vi "Double FFT Mesurament (Max Bin detection - Control - Windowing - DIEGO) test.vi"() -> ()   [LabVIEW 2014]
uses:
  <vilib>/Platform/TimedLoop/XDataNode/timing_clust.ctl
  <vilib>/Platform/TimedLoop/XDataNode/nitl_modes.ctl
  <vilib>/Platform/TimedLoop/XDataNode/wakeup.ctl
  <vilib>/rvi/Analysis/measure/FFT/simModelSupport/niFPGA FFT Streaming Sim Properties.ctl
  <vilib>/rvi/Analysis/measure/FFT/simModelSupport/niFPGA FFT Sim Stream Group Properties.ctl
  <vilib>/rvi/Analysis/measure/FFT/simModelSupport/niFPGA FFT Sim Types.ctl
  <vilib>/rvi/Analysis/measure/FFT/simModelSupport/niFpgaFFTSimArithmeticProperties.ctl
  <vilib>/rvi/Analysis/measure/FFT/simModelSupport/niFpgaFFTSimDfxp.ctl
  <vilib>/fxp/LVFixedPointQuantizationPolicyTypeDef.ctl
  <vilib>/rvi/Analysis/measure/FFT/XNode/niFpgaFFTButterflyDelays.ctl
  <vilib>/rvi/Emulation/niFpgaSctlEmulationGetInTimedLoop.vi
  <vilib>/rvi/Emulation/niFpgaEmulationReportErrorSimple.vi
  <vilib>/rvi/Emulation/niFpgaGetClockAttributes.vi
  <vilib>/rvi/Emulation/niFpgaCriticalErrorInLSC.vi
  <vilib>/rvi/Emulation/niFpgaEmulationIsFPGAContextNoSignature.vi
  <vilib>/rvi/errors/niFpgaSetErrorForExecOnDevCompSimple.vi
  <vilib>/rvi/eio/common/nirviEmuReportErrorAndStop.vi
  <vilib>/rvi/DataTransferAndStorage/Container/Common/niFpgaContainerGetUniqueNameForEmu.vi
  <vilib>/rvi/FIFO/Fifo_Resource/nirvififoEmulationSetSize.vi
  <vilib>/rvi/FIFO/Fifo_Resource/nirviFifoEmulationQueueMgr.vi
  <instcachedir>/0/nirviFifoEmulationQueueMgr_E5CAEC123FF24DC58D834DCA3CDAA9B5.lvgen/nirviFifoEmulationQueueMgr_E5CAEC123FF24DC58D834DCA3CDAA9B5_004.vi
  <vilib>/Utility/error.llb/Clear Errors.vi
  <vilib>/rvi/FIFO/Fifo_Resource/nirvififoEmulationCreateLock.vi
  <vilib>/rvi/Emulation/niFpgaProcessEmulError.vi
  <vilib>/rvi/FIFO/Fifo_Resource/nirvififoEmulationObtainLock.vi
  <vilib>/rvi/FIFO/Fifo_Resource/nirvififoEmulationReleaseLock.vi
  <vilib>/rvi/occurrence/nirviWaitOnOccurrenceBase.vi
  <vilib>/rvi/errors/nirviReportUnexpectedCaseInternalError.vi
  <vilib>/rvi/errors/nirviReportUnexpectedCaseInternalError (U32).vi
  <vilib>/rvi/Memory/Memory_Emulation/niFpgaMemoryEmulationCacheClearOnFirstRun.vi
  <vilib>/rvi/Memory/Memory_Emulation/nirvimemoryEmulationManagerCache_MakeExclusive.vi
  <vilib>/rvi/Memory/Memory_Emulation/niFpgaMemoryEmulationValidateCache.vi
  <vilib>/rvi/Memory/Memory_Emulation/nirvimemoryEmulationManagerCache_InsertValue.vi
  <vilib>/rvi/Memory/Memory_Emulation/nirvimemoryEmulationManagerCache_ReleaseExclusive.vi
  <vilib>/rvi/Memory/Memory_Emulation/nirvimemoryEmulationManagerCache_GetValue.vi
  <vilib>/rvi/Memory/Memory_Emulation/nirvimemoryEmulationManagerCache_SetValue.vi
  <instcachedir>/0/nirviFifoEmulationQueueMgr_E5CAEC123FF24DC58D834DCA3CDAA9B5.lvgen/nirviFifoEmulationQueueMgr_E5CAEC123FF24DC58D834DCA3CDAA9B5_003.vi
  <vilib>/rvi/FIFO/Fifo_Resource/nirvififoEmulationDetermineInputValidOut.vi
  <vilib>/rvi/Memory/Memory_Emulation/nirvimemoryFastEmulation.vi
  <vilib>/rvi/Memory/Memory_Emulation/nirvimemoryEmulation.vi
  <vilib>/rvi/interface/RandomDataEmulation/niFpgaRandomDataHandleErrors.vi
  <vilib>/rvi/Analysis/measure/FFT/simModelSupport/niFpgaFFTSimModelStreamingCore.vi
  <vilib>/rvi/eio/common/nirviEmuTemplateMethod_errors.vi
  <vilib>/Platform/TimedLoop/XDataNode/XDataNode.xnode
  <vilib>/rvi/DataTransferAndStorage/Container/XNode/niFpgaContainer.xnode
  <vilib>/rvi/FIFO/Fifo_Resource/nirvififoEmulationRead.vi
  <vilib>/rvi/DataTransferAndStorage/Register/Emulation/niFpgaRegisterEmulation.vi
  <vilib>/rvi/FIFO/Fifo_Resource/nirvififoEmulationWrite.vi
  <vilib>/rvi/FIFO/Fifo_Resource/nirvififoEmulationGetNumberOfElementsToWrite.vi
  <vilib>/rvi/interface/RandomDataEmulation/nirviRandomDataFpgaReadWriteTemplate.vi
  <vilib>/rvi/Analysis/measure/FFT/XNode/niFpgaFFT.xnode
  <vilib>/eio/EIOMethodNode/EIOMethodNode.xnode
  <vilib>/Platform/TimedLoop/XDataNode/XDNodeRunTimeDep.lvlib
panel:
  in  "snapshot":bool
  in  "first bin":i32=4
  in  "last bin":i32=251
  in  "lower limit 2":u32=682
  in  "lower limit 1":u32=57
  in  "upper limit 2":u32=1194
  in  "upper limit 1":u32=569
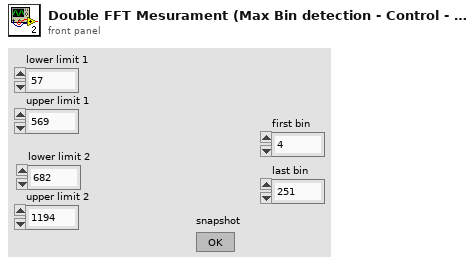
[diagram p1: front panel]
types:
  T1 = typedef "XDNodeRunTimeDep.lvlib/timing_clust.ctl" = cluster{"Expected End [f-1]":u64, "Actual End [f-1]":u64, "Finished Late? [f-1]":bool, "Expected End [i-1]":u64, "Actual End [i-1]":u64, "Finished Late? [i-1]":bool, "Expected Start [i]":u64, "Actual Start [i]":u64, "Expected Start [f]":u64, "Actual Start [f]":u64, "Source Name":string, "Structure Name":string, "Period":i64, "Deadline":i64, "Offset":i64, "Start":i64, "Priority":i32, "Timeout":i32, "Mode":T2, "Wakeup Reason":T3, "Error":errorcluster, "Source Type":string, "Secondary Source Type":string, "Global End Time":u64, "Global Start Time":u64, "Frame Duration":u64, "Iteration Duration":u64, "Assigned CPU":i32, "I/O Scan Engine Mode":u32}
  T2 = typedef "XDNodeRunTimeDep.lvlib/nitl_modes.ctl" = enum32{"No Change", "Process missed periods, maintain original phase", "Discard missed periods, maintain original phase", "Process missed periods, ignore original phase", "Discard missed periods, ignore original phase"}
  T3 = typedef "XDNodeRunTimeDep.lvlib/wakeup.ctl" = enum32{"Normal", "Aborted", "Asynchronous wakeup", "Timing source error", "Timed loop error", "Timeout"}
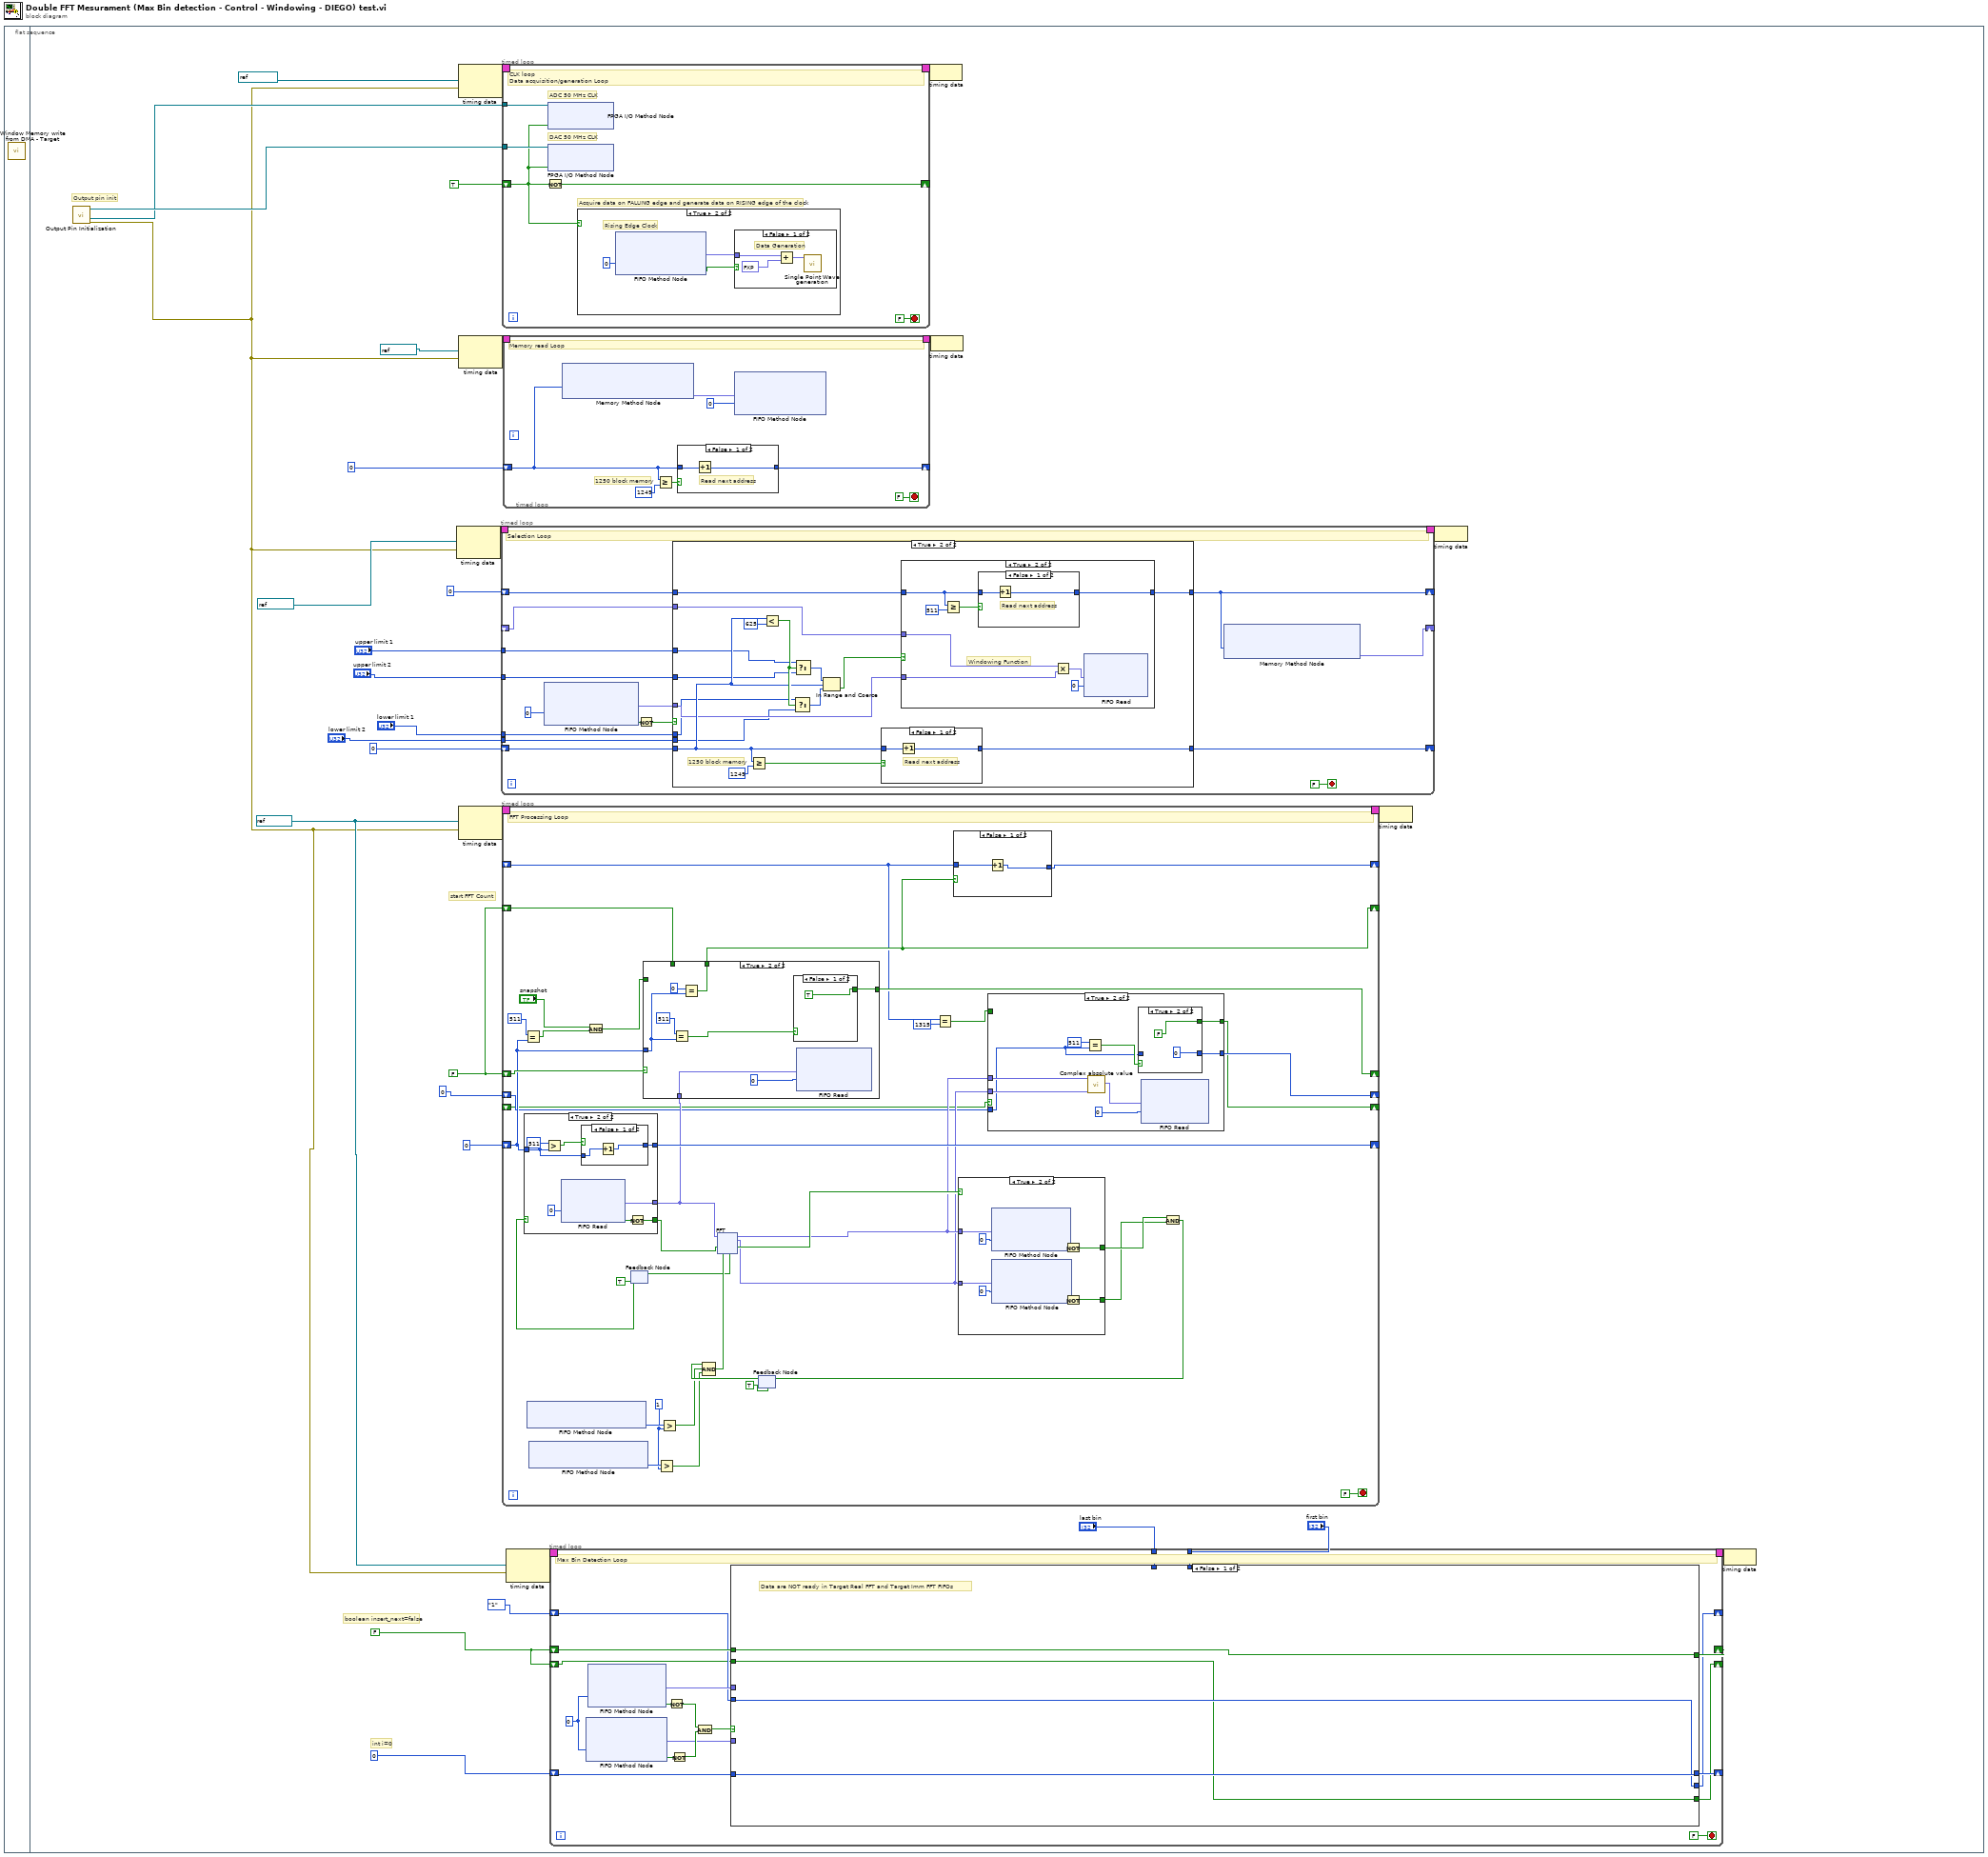
[diagram p0: block diagram]
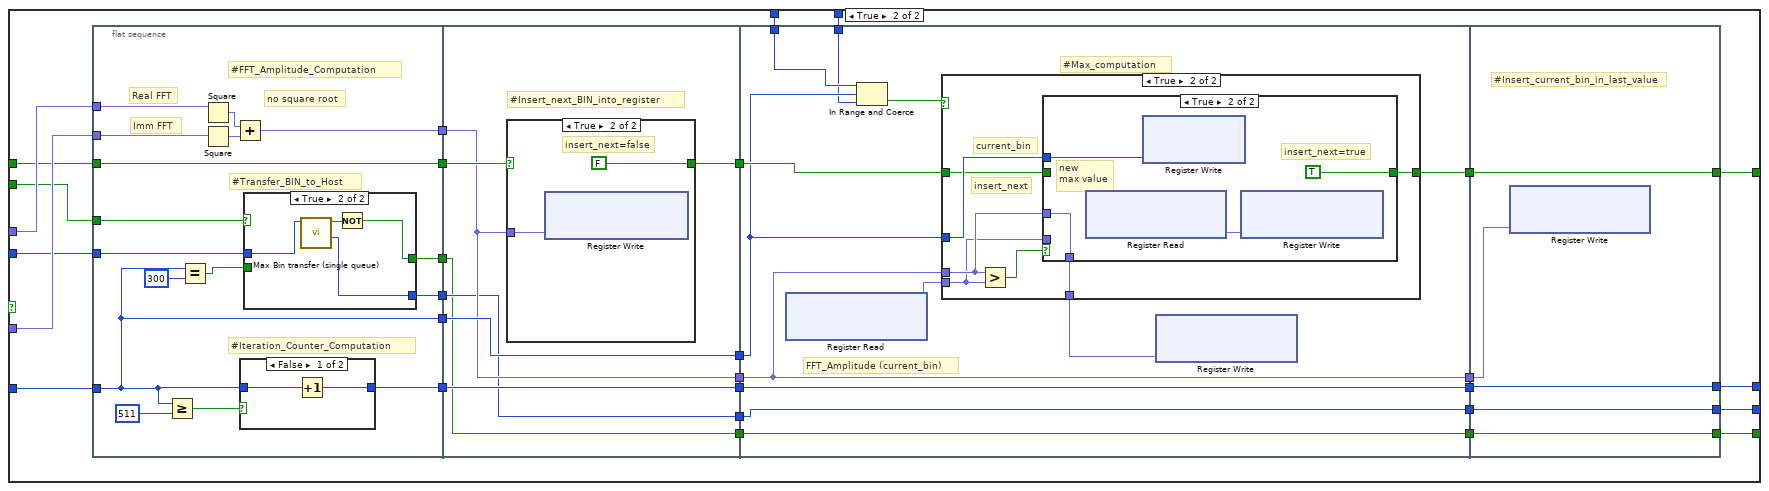
[diagram p2: hidden frame]
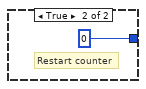
[diagram p4: hidden frame]
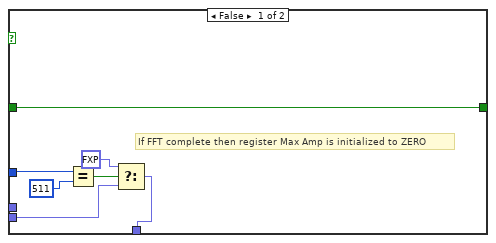
[diagram p6: hidden frame]
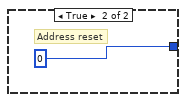
[diagram p10: hidden frame]
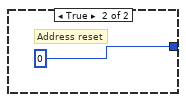
[diagram p11: hidden frame]
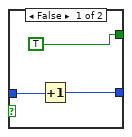
[diagram p13: hidden frame]
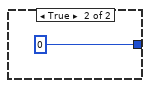
[diagram p14: hidden frame]
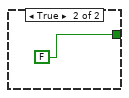
[diagram p16: hidden frame]
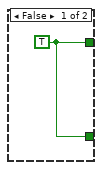
[diagram p17: hidden frame]
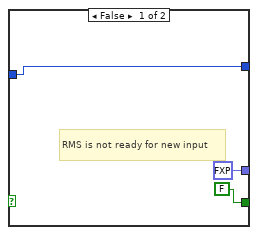
[diagram p18: hidden frame]
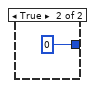
[diagram p19: hidden frame]
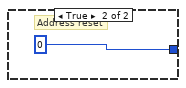
[diagram p20: hidden frame]
diagram:
  n1 = flat-sequence {
    frame #0 {
      n2 = call "Window Memory write from DMA - Target.vi"() -> ()  [unwired: 12 in]
    }
    frame #1 {
      w4 = FALSE
      w1 = FALSE
      w14 = refnum<k21> "50MHz" ("Source Name")
      # "start FFT Count"
      # "int i=0"
      # "boolean insert_next=false"
      # "Output pin init"
      n3 = call "Output Pin Initialization.vi"() -> ("error out"=w13:errorcluster, "I/O Out Clock DAC (pin16)"=w18:refnum<k21>, "I/O Out Clock ADC (pin17)"=w19:refnum<k21>)  [unwired: 8 in]
      n4 = node-c288(refnum<k21> "50MHz" ("Source Name"), w13) -> (w27:T1)
      n5 = node-c288(refnum<k21> "100MHz" ("Source Name"), w13) -> (w33:T1)
      n6 = node-c288(w14, w13) -> (w29:T1)
      n7 = node-c288(refnum<k21> "50MHz" ("Source Name"), w13) -> (w31:T1)
      n8 = timed-loop {
        timing: w27 -> [_]
        timing-out: [_] -> w26
        shift-right: [w178] -> _
        shift-left: u32 0 -> [w177]
        tunnel: "upper limit 1" -> [w172]
        tunnel: "upper limit 2" -> [w171]
        tunnel: "lower limit 1" -> [w170]
        tunnel: "lower limit 2" -> [w169]
        shift-right: [w165] -> _
        shift-left: u32 0 -> [w168]
        shift-right: [w166] -> _
        shift-left: _ -> [w167]
        stop <- FALSE stop-if-true
        # "Selection Loop"
        n9 = xnode ("FIFO Method Node")("Timeout"=0) -> ("Element"=w174:fxp<+/-,12,12>, "Timed Out?"=w175:bool)  [unwired: 1 in, 1 out]
        n10 = Not(x=w175) -> (.not. x?=w176:bool)
        n11 = case shown="True" w176 {
          tunnel: [w181 w196] -> w178
          tunnel: w177 -> [w181 w191]
          tunnel: w174 -> [_ w189]
          tunnel: w172 -> [_ w188]
          tunnel: w171 -> [_ w187]
          tunnel: w170 -> [_ w186]
          tunnel: w169 -> [_ w185]
          tunnel: w168 -> [w180 w182]
          tunnel: [w180 w184] -> w165
          tunnel: w167 -> [_ w183]
          frame False {
          }
          frame True {
            # "1250 block memory"
            n12 = Greater Or Equal?(x=w191, y=u32 1249) -> (x >= y?=w197:bool)
            n13 = Less?(x=w191, y=u32 625) -> (x < y?=w192:bool)
            n14 = Select(t=w186, s=w192, f=w185) -> (s? t:f=w194:u32)
            n15 = Select(t=w188, s=w192, f=w187) -> (s? t:f=w195:u32)
            n16 = In Range and Coerce(upper limit=w195, x=w191, lower limit=w194) -> (In Range?=w190:bool)  [unwired: 1 out]
            n17 = case shown="False" w197 {
              tunnel: w191 -> [w212 _]
              tunnel: [w211 u32 0] -> w196
              frame False {
                # "Read next address"
                n18 = Increment(x=w212) -> (x+1=w211:u32)
              }
              frame True {
                # "Address reset"
              }
            }
            n19 = case shown="True" w190 {
              tunnel: w189 -> [_ w206]
              tunnel: w182 -> [w199 w202]
              tunnel: [w199 w204] -> w184
              tunnel: w183 -> [_ w200]
              frame False {
              }
              frame True {
                # "Windowing Function"
                n20 = Greater Or Equal?(x=w202, y=u32 511) -> (x >= y?=w203:bool)
                n21 = case shown="False" w203 {
                  tunnel: w202 -> [w209 _]
                  tunnel: [w208 u32 0] -> w204
                  frame False {
                    # "Read next address"
                    n22 = Increment(x=w209) -> (x+1=w208:u32)
                  }
                  frame True {
                    # "Address reset"
                  }
                }
                n23 = Multiply(x=w200, y=w206) -> (x*y=w205:fxp<+/-,12,12>)
                n24 = xnode ("FIFO Read")("Element"=w205, "Timeout"=0) -> ()  [unwired: 1 in, 2 out]
              }
            }
          }
        }
        n25 = xnode ("Memory Method Node")("Address"=w165) -> ("Data"=w166:fxp<+,8,1>)  [unwired: 1 in, 1 out]
      }
      n26 = timed-loop {
        timing: w33 -> [_]
        timing-out: [_] -> w32
        shift-right: [w365] -> _
        shift-left: TRUE -> [w363]
        tunnel: w18 -> [w367]
        tunnel: w19 -> [w364]
        stop <- FALSE stop-if-true
        # "DAC 50 MHz CLK"
        # "Acquire data on FALLING edge and generate data on RISING edge of the clock"
        # "ADC 50 MHz CLK"
        # "CLK loop\nData acquisition/generation Loop"
        n27 = Not(x=w363) -> (.not. x?=w365:bool)
        n28 = xnode "FPGA I/O Method Node"("FPGA I/O In"=w367, "Data"=w363) -> ()  [unwired: 1 out]
        n29 = xnode "FPGA I/O Method Node"("FPGA I/O In"=w364, "Data"=w363) -> ()  [unwired: 1 out]
        n30 = case shown="True" w363 {
          frame False {
            # "Falling Edge Clock"
            n31 = call "Single Acquisition.vi"() -> ("Out"=w369:fxp<+/-,12,12>)  [unwired: 10 in, 1 out]
            n32 = xnode ("FIFO Method Node")("Element"=w369, "Timeout"=0) -> ()  [unwired: 1 in, 2 out]
          }
          frame True {
            # "Rising Edge Clock"
            n33 = xnode ("FIFO Method Node")("Timeout"=0) -> ("Element"=w370:fxp<+/-,12,12>, "Timed Out?"=w371:bool)  [unwired: 1 in, 1 out]
            n34 = case shown="False" w371 {
              tunnel: w370 -> [w375 _]
              frame False {
                # "Data Generation"
                n35 = Add(x=w375, y=fxp<+,12,12> 2048.0) -> (x+y=w373:fxp<+/-,14,14>)
                n36 = call "Single Point Wave generation.vi"("Data To Write"=w373) -> ()  [unwired: 10 in, 1 out]
              }
              frame True {
                # "FPGA memory slow"
              }
            }
          }
        }
      }
      n37 = timed-loop {
        timing: w29 -> [_]
        timing-out: [_] -> w28
        shift-right: [w241] -> _
        shift-left: 0 ("Timeout") -> [w233]
        shift-right: [w236] -> _
        shift-left: w4 -> [w235]
        shift-right: [w231] -> _
        shift-left: w4 -> [w232]
        shift-right: [w230] -> _
        shift-left: _ -> [w229]
        shift-right: [w223] -> _
        shift-left: i16 0 -> [w224]
        shift-right: [w222] -> _
        shift-left: _ -> [w221]
        stop <- FALSE stop-if-true
        w244 = u32 1 ("y")
        # "FFT Processing Loop"
        n38 = Equal?(x=511, y=w233) -> (x = y?=w239:bool)
        n39 = xnode ("FIFO Method Node")() -> ("Number of Elements to Write"=w246:u32)  [unwired: 1 in, 1 out]
        n40 = xnode ("FIFO Method Node")() -> ("Number of Elements to Write"=w245:u32)  [unwired: 1 in, 1 out]
        n41 = And(x="snapshot", y=w239) -> (x .and. y?=w237:bool)
        n42 = feedback #1(TRUE ("ready for input")) -> (w258:bool)
        n43 = case shown="True" w258 {
          tunnel: [FALSE w335] -> w253
          tunnel: [fxp<+/-,12,12> 0.0 ("Element") w332] -> w234
          tunnel: w233 -> [w325 w328]
          tunnel: [w325 w329] -> w241
          frame False {
            # "RMS is not ready for new input"
          }
          frame True {
            n44 = Greater?(x=511, y=w328) -> (0:w330:bool)
            n45 = xnode ("FIFO Read")("Timeout"=0) -> ("Element"=w332:fxp<+/-,12,12>, "Timed Out?"=w334:bool)  [unwired: 1 in, 1 out]
            n46 = case shown="False" w330 {
              tunnel: [w336 0 ("Timeout")] -> w329
              tunnel: w328 -> [w337 _]
              frame False {
                n47 = Increment(x=w337) -> (x+1=w336:i32)
              }
              frame True {
              }
            }
            n48 = Not(x=w334) -> (.not. x?=w335:bool)
          }
        }
        n49 = case shown="True" w235 {
          tunnel: w237 -> [w279 _]
          tunnel: [w279 w283] -> w236
          tunnel: w234 -> [_ w287]
          tunnel: w233 -> [_ w282]
          tunnel: [w278 w281] -> w231
          tunnel: w232 -> [w278 _]
          frame False {
          }
          frame True {
            n50 = Equal?(x=511, y=w282) -> (x = y?=w284:bool)
            n51 = Equal?(x=0, y=w282) -> (x = y?=w281:bool)
            n52 = case shown="False" w284 {
              tunnel: [TRUE FALSE] -> w283
              frame False {
              }
              frame True {
              }
            }
            n53 = xnode ("FIFO Read")("Element"=w287, "Timeout"=0) -> ()  [unwired: 1 in, 2 out]
          }
        }
        n54 = Greater?(x=w245, y=w244) -> (0:w242:bool)
        n55 = Greater?(x=w246, y=w244) -> (0:w243:bool)
        n56 = feedback #2(TRUE) -> (w254:bool)
        n57 = Compound Arithmetic op=AND(w254, w243, w242) -> (w252:bool)
        n58 = xnode "FFT"("real data in"=w234, "input valid"=w253, "ready for output"=w252) -> ("ready for input"=w251:bool, "real data out"=w226:fxp<+/-,22,22>, "imaginary data out"=w225:fxp<+/-,22,22>, "output valid"=w250:bool)  [unwired: 2 in, 1 out]
        n59 = feedback-in #1(w251) -> ()
        n60 = Equal?(x=w229, y=1315) -> (x = y?=w227:bool)
        n61 = case shown="False" w231 {
          tunnel: [w275 0 ("x")] -> w230
          tunnel: w229 -> [w276 _]
          frame False {
            n62 = Increment(x=w276) -> (x+1=w275:i32)
          }
          frame True {
          }
        }
        n63 = case shown="True" w250 {
          tunnel: w226 -> [_ w324]
          tunnel: w225 -> [_ w323]
          tunnel: [w316 w322] -> w249
          tunnel: [w316 w321] -> w248
          frame False {
            w316 = TRUE
          }
          frame True {
            n64 = xnode ("FIFO Method Node")("Element"=w324, "Timeout"=0) -> ("Timed Out?"=w317:bool)  [unwired: 1 in, 1 out]
            n65 = xnode ("FIFO Method Node")("Element"=w323, "Timeout"=0) -> ("Timed Out?"=w318:bool)  [unwired: 1 in, 1 out]
            n66 = Not(x=w317) -> (.not. x?=w322:bool)
            n67 = Not(x=w318) -> (.not. x?=w321:bool)
          }
        }
        n68 = case shown="True" w221 {
          tunnel: w227 -> [w260 _]
          tunnel: [w260 w268] -> w222
          tunnel: w226 -> [_ w266]
          tunnel: w225 -> [_ w265]
          tunnel: w224 -> [w259 w262]
          tunnel: [w259 w261] -> w223
          frame False {
          }
          frame True {
            n69 = Equal?(x=i16 511, y=w262) -> (x = y?=w264:bool)
            n70 = call "Complex absolute value.vi"("Im"=w265, "Re"=w266) -> ("Square Absolute Value"=w267:fxp<+,44,44>)  [unwired: 9 in]
            n71 = case shown="True" w264 {
              tunnel: [TRUE FALSE] -> w268
              tunnel: w262 -> [w271 _]
              tunnel: [w270 i16 0 ("x")] -> w261
              frame False {
                n72 = Increment(x=w271) -> (x+1=w270:i16)
              }
              frame True {
              }
            }
            n73 = xnode ("FIFO Read")("Element"=w267, "Timeout"=0) -> ()  [unwired: 1 in, 2 out]
          }
        }
        n74 = Compound Arithmetic op=AND(w249, w248) -> (w247:bool)
        n75 = feedback-in #2(w247) -> ()
      }
      n76 = timed-loop {
        timing: w31 -> [_]
        timing-out: [_] -> w30
        shift-right: [w350] -> _
        shift-left: u32 0 -> [w348]
        stop <- FALSE stop-if-true
        # "1250 block memory"
        # "Memory read Loop"
        n77 = xnode ("Memory Method Node")("Address"=w348) -> ("Data"=w347:fxp<+/-,12,12>)  [unwired: 1 in, 1 out]
        n78 = Greater Or Equal?(x=w348, y=u32 1249) -> (x >= y?=w351:bool)
        n79 = case shown="False" w351 {
          tunnel: w348 -> [w354 _]
          tunnel: [w353 u32 0] -> w350
          frame False {
            # "Read next address"
            n80 = Increment(x=w354) -> (x+1=w353:u32)
          }
          frame True {
            # "Address reset"
          }
        }
        n81 = xnode ("FIFO Method Node")("Element"=w347, "Timeout"=0) -> ()  [unwired: 1 in, 2 out]
      }
      n82 = node-c288(w14, w13) -> (w25:T1)
      n83 = timed-loop {
        shift-right: [w43] -> _
        shift-left: 0 ("Timeout") -> [w44]
        shift-right: [w41] -> _
        shift-left: w1 -> [w42]
        timing: w25 -> [_]
        timing-out: [_] -> w24
        tunnel: "last bin" -> [w39]
        tunnel: "first bin" -> [w38]
        shift-right: [w36] -> _
        shift-left: enum16{"1", "2", "3", "4"}."1" ("Enum") -> [w37]
        shift-right: [w34] -> _
        shift-left: w1 -> [w35]
        stop <- FALSE stop-if-true
        w52 = 0 ("Timeout")
        # "Max Bin Detection Loop"
        n84 = xnode ("FIFO Method Node")("Timeout"=w52) -> ("Element"=w45:fxp<+/-,22,22>, "Timed Out?"=w50:bool)  [unwired: 1 in, 1 out]
        n85 = xnode ("FIFO Method Node")("Timeout"=w52) -> ("Element"=w46:fxp<+/-,22,22>, "Timed Out?"=w51:bool)  [unwired: 1 in, 1 out]
        n86 = Not(x=w51) -> (.not. x?=w49:bool)
        n87 = Not(x=w50) -> (.not. x?=w48:bool)
        n88 = And(x=w49, y=w48) -> (x .and. y?=w47:bool)
        n89 = case shown="False" w47 {
          tunnel: w46 -> [_ w85]
          tunnel: w45 -> [_ w84]
          tunnel: w44 -> [w56 w82]
          tunnel: [w56 w69] -> w43
          tunnel: w42 -> [w55 w76]
          tunnel: [w55 w71] -> w41
          tunnel: w39 -> [_ w68]
          tunnel: w38 -> [_ w67]
          tunnel: w37 -> [w54 w66]
          tunnel: [w54 w62] -> w36
          tunnel: w35 -> [w53 w61]
          tunnel: [w53 w60] -> w34
          frame False {
            # "Data are NOT ready in Target Real FFT and Target Imm FFT FIFOs"
          }
          frame True {
            n90 = flat-sequence {
              tunnel: w85 -> [w98]
              tunnel: w84 -> [w99]
              tunnel: [w97] -> w83
              tunnel: w82 -> [w91]
              tunnel: [w96] -> w81
              tunnel: [w91] -> w78
              tunnel: [w93] -> w77
              tunnel: w76 -> [w93]
              tunnel: w66 -> [w90]
              tunnel: [w89] -> w64
              tunnel: w61 -> [w87]
              tunnel: [w86] -> w57
              tunnel: w83 -> [w114]
              tunnel: w81 -> [w117]
              tunnel: [w117] -> w80
              tunnel: w78 -> [w115]
              tunnel: w77 -> [w116]
              tunnel: [w115] -> w75
              tunnel: [w114] -> w74
              tunnel: [w113] -> w73
              tunnel: [w112] -> w65
              tunnel: w64 -> [w112]
              tunnel: [w111] -> w58
              tunnel: w57 -> [w111]
              tunnel: w80 -> [w132]
              tunnel: [w132] -> w79
              tunnel: w75 -> [w127]
              tunnel: w74 -> [w129]
              tunnel: w73 -> [w130]
              tunnel: [w129] -> w72
              tunnel: [w128] -> w70
              tunnel: w68 -> [w124]
              tunnel: w67 -> [w123]
              tunnel: w65 -> [w122]
              tunnel: [w122] -> w63
              tunnel: [w121] -> w59
              tunnel: w58 -> [w121]
              tunnel: w79 -> [w155]
              tunnel: w72 -> [w157]
              tunnel: w70 -> [w156]
              tunnel: [w156] -> w71
              tunnel: [w155] -> w69
              tunnel: [w154] -> w62
              tunnel: w63 -> [w154]
              tunnel: [w153] -> w60
              tunnel: w59 -> [w153]
              frame #0 {
                # "no square root"
                # "#Transfer_BIN_to_Host"
                # "#Iteration_Counter_Computation"
                # "#FFT_Amplitude_Computation"
                # "Imm FFT"
                # "Real FFT"
                n91 = Greater Or Equal?(x=w91, y=511) -> (x >= y?=w94:bool)
                n92 = Equal?(x=w91, y=300) -> (x = y?=w88:bool)
                n93 = Square(x=w98) -> (x^2=w101:fxp<+,43,43>)
                n94 = Square(x=w99) -> (x^2=w100:fxp<+,43,43>)
                n95 = Add(x=w101, y=w100) -> (x+y=w97:fxp<+,44,44>)
                n96 = case shown="False" w94 {
                  tunnel: w91 -> [w108 _]
                  tunnel: [w109 0 ("Timeout")] -> w96
                  frame False {
                    n97 = Increment(x=w108) -> (x+1=w109:i32)
                  }
                  frame True {
                    # "Restart counter"
                  }
                }
                n98 = case shown="True" w87 {
                  tunnel: w88 -> [w103 _]
                  tunnel: [w103 w106] -> w86
                  tunnel: w90 -> [w102 w105]
                  tunnel: [w102 w104] -> w89
                  frame False {
                    # "FFT Comp is NOT finished"
                  }
                  frame True {
                    n99 = call "Max Bin transfer (single queue).vi"("Enum"=w105) -> ("Next state"=w104:enum16{"1", "2", "3", "4"}, "END?"=w107:bool)  [unwired: 9 in]
                    n100 = Not(x=w107) -> (.not. x?=w106:bool)
                  }
                }
              }
              frame #1 {
                # "#Insert_next_BIN_into_register"
                n101 = case shown="True" w116 {
                  selector: w116 -> [w118 _]
                  tunnel: [w118 FALSE] -> w113
                  tunnel: w114 -> [_ w119]
                  frame False {
                  }
                  frame True {
                    # "insert_next=false"
                    n102 = xnode ("Register Write")("Data"=w119) -> ()  [unwired: 1 in, 1 out]
                  }
                }
              }
              frame #2 {
                # "FFT_Amplitude (current_bin)"
                # "#Max_computation"
                n103 = xnode ("Register Read")() -> ("Data"=w126:fxp<+,44,44>)  [unwired: 1 in, 1 out]
                n104 = In Range and Coerce(upper limit=w124, x=w127, lower limit=w123) -> (In Range?=w131:bool)  [unwired: 1 out]
                n105 = case shown="True" w131 {
                  tunnel: w129 -> [_ w145]
                  tunnel: w127 -> [w137 w144]
                  tunnel: w130 -> [w139 w143]
                  tunnel: [w139 w142] -> w128
                  tunnel: w126 -> [w135 w140]
                  tunnel: [w133 w141] -> w125
                  frame False {
                    # "If FFT complete then register Max Amp is initialized to ZERO"
                    n106 = Equal?(x=w137, y=511) -> (x = y?=w138:bool)
                    n107 = Select(t=fxp<+,44,44> 0.0, s=w138, f=w135) -> (s? t:f=w133:fxp<+,44,44>)
                  }
                  frame True {
                    # "insert_next"
                    # "current_bin"
                    n108 = Greater?(x=w145, y=w140) -> (0:w146:bool)
                    n109 = case shown="True" w146 {
                      tunnel: w145 -> [_ w149]
                      tunnel: w144 -> [_ w152]
                      tunnel: w143 -> [w148 _]
                      tunnel: [w148 TRUE] -> w142
                      tunnel: [w147 w149] -> w141
                      tunnel: w140 -> [w147 _]
                      frame False {
                        # "Old value is re-written"
                      }
                      frame True {
                        # "new\nmax value"
                        # "insert_next=true"
                        n110 = xnode ("Register Read")() -> ("Data"=w150:fxp<+,44,44>)  [unwired: 1 in, 1 out]
                        n111 = xnode ("Register Write")("Data"=w152) -> ()  [unwired: 1 in, 1 out]
                        n112 = xnode ("Register Write")("Data"=w150) -> ()  [unwired: 1 in, 1 out]
                      }
                    }
                  }
                }
                n113 = xnode ("Register Write")("Data"=w125) -> ()  [unwired: 1 in, 1 out]
              }
              frame #3 {
                # "#Insert_current_bin_in_last_value"
                n114 = xnode ("Register Write")("Data"=w157) -> ()  [unwired: 1 in, 1 out]
              }
            }
          }
        }
      }
      n115 = node-c288(w32) -> ()
      n116 = node-c288(w30) -> ()
      n117 = node-c288(w28) -> ()
      n118 = node-c288(w26) -> ()
      n119 = node-c288(w24) -> ()
    }
  }
